vi "三角波子vi.vi"(10 "幅值":dbl) -> (3 "数组":dbl[](array[numeric]))   [LabVIEW 2018]
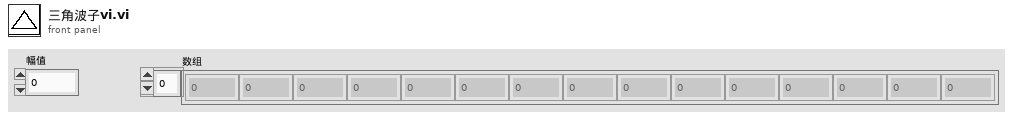
[diagram p1: front panel]
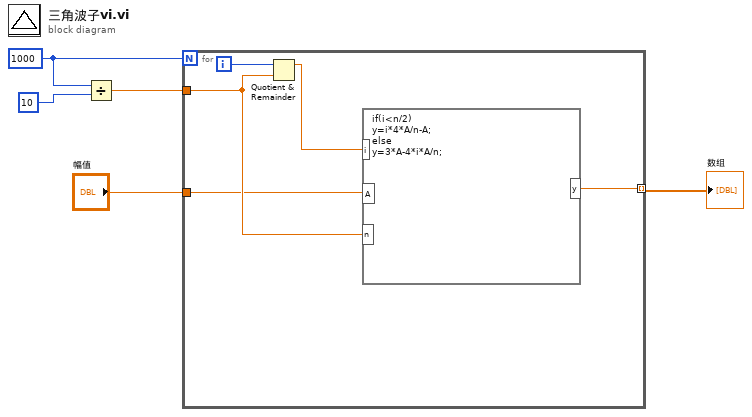
[diagram p0: block diagram]
diagram:
  w4 = 1000
  n1 = Divide(x=w4, y=10) -> (x/y=w3:dbl)
  n2 = for {
    N: w4 -> [_]
    tunnel: w3 -> [w8]
    tunnel: "幅值" -> [w7]
    tunnel: [w6] -> w1 mode=indexing
    i -> [w10]
    n3 = Quotient & Remainder(x=w10, y=w8) -> (x-y*floor(x/y)=w9:dbl)  [unwired: 1 out]
    n4 = formula code="if(i<n/2)\ny=i*4*A/n-A;\nelse\ny=3*A-4*i*A/n;"("i"=w9, "A"=w7, "n"=w8) -> ("y"=w6:dbl)
  }
  "数组" <- w1
